vi "myANPR Host PC.vi"() -> ()   [LabVIEW 2014]
doc: "This is the Host PC VI to the myANPR system. An array of strings is passed through a network published shared variable to this VI which logs all the strings to a file in My Documents under the name 'myANPR<date>'.txt."
uses:
  <vilib>/Utility/sysdir.llb/System Directory Type.ctl
panel:
  out "myANPR":string[](array[string])
  in  "Stop Button":bool
  # "All data collected by the myANPR system\nis logged to a text file in the corresponding\nDocuments folder titled the date"
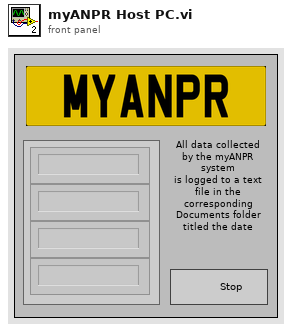
[diagram p1: front panel]
types:
  T1 = enum16{"open", "replace", "create", "open or create", "replace or create", "replace or create with confirmation"}
  T2 = typedef "System Directory Type.ctl" = i32
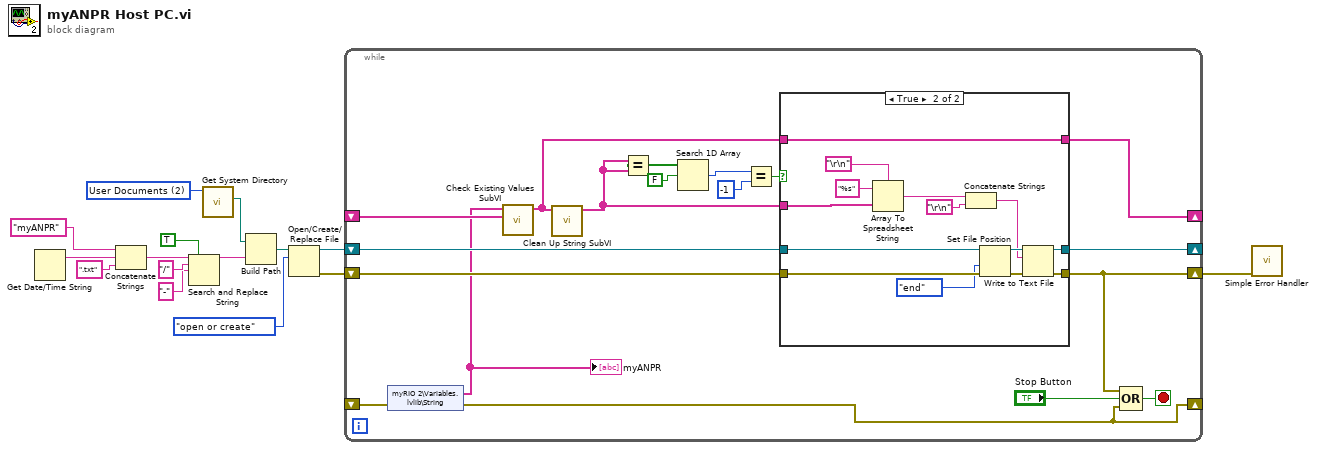
[diagram p0: block diagram]
diagram:
  w15 = T2 2 items=["User Home"=0, "User Desktop"=1, "User Documents"=2, "User Application Data"=3, "User Preferences"=4, "User Temporary"=5, "Public Documents"=6, "Public Application Data"=7, "Public Preferences"=8, "Public Cache"=13, "System Core Libraries"=9, "System Installed Libraries"=10, "Application Files"=11, "Boot Volume Root"=12] ("system directory type")
  n1 = Get Date/Time String() -> (date string=w13:string)  [unwired: 3 in, 1 out]
  n2 = Concatenate Strings("myANPR" ("name or relative path"), w13, ".txt" ("string")) -> (w11:string)
  n3 = Search and Replace String(replace all?=TRUE ("replace all? (F)"), input string=w11, search string="/", replace string="-" ("replace string (\"\")")) -> (result string=w5:string)  [unwired: 4 in, 3 out]
  n4 = call <vilib>:"Get System Directory.vi"("system directory type"=w15) -> ("system directory"=w14:path)  [unwired: 10 in]
  n5 = Build Path(base path=w14, name or relative path=w5) -> (appended path=w7:path)
  n6 = Open/Create/Replace File(file path (use dialog)=w7, operation (0:open)=T1."open or create") -> (refnum out=w2:refnum<file>, error out=w1:errorcluster)  [unwired: 4 in, 1 out]
  n7 = while {
    shift-right: [w31] -> _
    shift-left: w2 -> [w33]
    shift-right: [w26] -> w3
    shift-left: w1 -> [w32]
    shift-right: [w27] -> _
    shift-left: _ -> [w30]
    shift-right: [w25] -> _
    shift-left: _ -> [w24]
    stop <- w29 stop-if-true
    n8 = shared-variable "myRIO 2\\Variables.lvlib\\String"(error in=w30) -> (w23:string[], error out=w27:errorcluster)
    "myANPR" <- w23
    n9 = call "Check Existing Values SubVI.vi"("Previous Value"=w24, "String Array from Variable"=w23) -> ("String Array"=w22:string[])  [unwired: 9 in]
    n10 = call "Clean Up String SubVI.vi"("String from OCR"=w22) -> ("Cleaned Up String"=w16:string[])  [unwired: 10 in]
    n11 = Equal?(x=w16, y=w16) -> (x = y?=w19:bool[])
    n12 = Search 1D Array(1D array=w19, element=FALSE) -> (index of element=w21:i32)  [unwired: 1 in]
    n13 = Equal?(x=w21, y=-1) -> (x = y?=w17:bool)
    n14 = case shown="True" w17 {
      tunnel: w33 -> [w36 w50]
      tunnel: w32 -> [w35 w49]
      tunnel: [w36 w48] -> w31
      tunnel: w16 -> [_ w39]
      tunnel: [w35 w38] -> w26
      tunnel: w22 -> [w34 w37]
      tunnel: [w34 w37] -> w25
      frame False {
      }
      frame True {
        n15 = Array To Spreadsheet String(delimiter (Tab)="\r\n", array=w39, 3:"%s" ("format string")) -> (spreadsheet string=w42:string)
        n16 = Concatenate Strings(w42, "\r\n") -> (w43:string)
        n17 = Set File Position(refnum=w50, from (0:start)=enum16{"start", "end", "current"}."end", error in=w49) -> (refnum out=w46:refnum<file>, error out=w47:errorcluster)  [unwired: 1 in]
        n18 = Write to Text File(file (use dialog)=w46, text=w43, error in=w47) -> (refnum out=w48:refnum<file>, error out=w38:errorcluster)  [unwired: 1 in, 1 out]
      }
    }
    n19 = Compound Arithmetic op=OR(w26, "Stop Button", w27) -> (w29:bool)
  }
  n20 = call <vilib>:"Simple Error Handler.vi"("error in (no error)"=w3) -> ()  [unwired: 4 in, 5 out]
